vi "Write COM.vi"(8 "error in (no error)":errorcluster, 10 "COM":refnum<visa-resource-name>, 11 "Tektronic in":refnum<class "Tektronic.lvclass">) -> (0 "error out":errorcluster, 3 "Tektronic out":refnum<class "Tektronic.lvclass">)   [LabVIEW 2020, in "Controlador.lvlib" / "Tektronic.lvclass"]
uses:
  Tektronic/Tektronic.lvclass
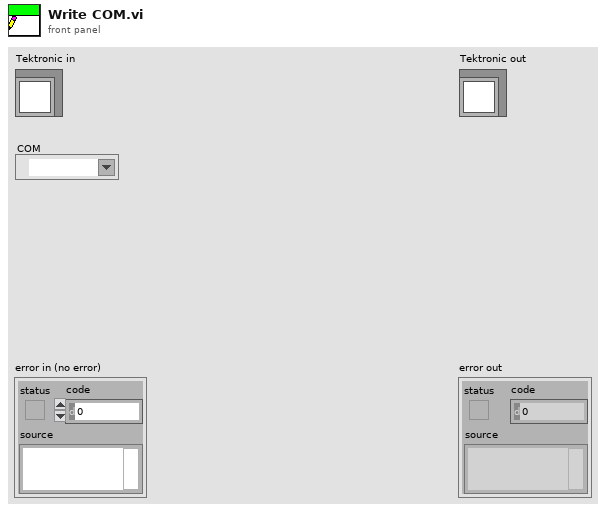
[diagram p1: front panel]
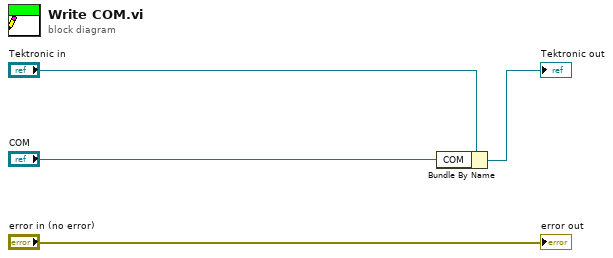
[diagram p0: block diagram]
diagram:
  n1 = Bundle By Name(cluster="Tektronic in", "COM"="COM") -> (→"Tektronic out":refnum<class "Tektronic.lvclass">)
  "error out" <- "error in (no error)"
